vi "Example - Caller is not JKISM++.vi"() -> ()   [LabVIEW 2014]
uses:
  user.lib/_NEVSTOP/JKI State Machine++/AdvanceAPI/CSM - Global Log Event.vi
  user.lib/_NEVSTOP/JKI State Machine++/_Support/JKISMQ/_CSMQFGV.vi
  user.lib/_NEVSTOP/JKI State Machine++/_Support/GlobalEvent/FGV-GlobalEventRef.vi
  user.lib/_NEVSTOP/JKI State Machine++/Communicable State Machine.lvlib
panel:
  in  "Log":bool
  out "Name":string[](array[string])
  in  "DoSth: DoC(error)":bool
  in  "DoSth: DoB":bool
  in  "DoSth: DoA":bool
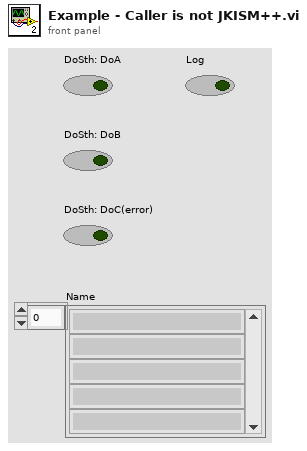
[diagram p1: front panel]
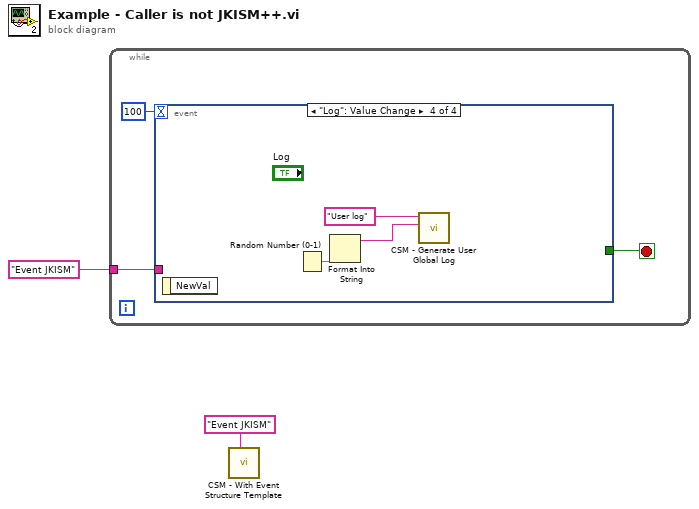
[diagram p0: block diagram]
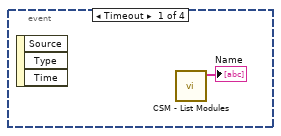
[diagram p2: hidden frame]
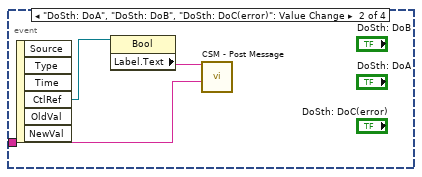
[diagram p3: hidden frame]
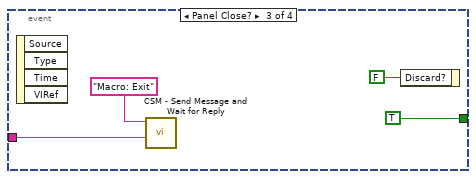
[diagram p4: hidden frame]
diagram:
  n1 = while {
    tunnel: "Event JKISM" ("Name(\"\" to use uuid)") -> [w4]
    stop <- w5 stop-if-true
    n2 = event shown="[3] \"Log\": Value Change" {
      selector: _ -> [_ _ _ _]
      dyn-events: _ -> [_ _ _ _]
      timeout: 100 -> [_ _ _ _]
      tunnel: [_ _ TRUE ("Discard?") _] -> w5
      tunnel: w4 -> [_ w9 w10 _]
      event Timeout {
        n3 = event-data() -> ()  [unwired: 1 in, 3 out]
        n4 = call "CSM - List Modules.vi"() -> ("Module Names"=→"Name":string[])  [unwired: 10 in, 1 out]
      }
      event "DoSth: DoA", "DoSth: DoB", "DoSth: DoC(error)": Value Change {
        n5 = event-data() -> ("CtlRef"=w8:refnum<vi>)  [unwired: 1 in, 5 out]
        n6 = property class="Bool"(reference=w8) -> ("Label.Text"=w7:string)  [unwired: 1 in, 2 out]
        n7 = call "CSM - Post Message.vi"("Target Module"=w9, "State"=w7) -> ()  [unwired: 9 in, 1 out]
      }
      event Panel Close? {
        n8 = event-data() -> ()  [unwired: 1 in, 4 out]
        n9 = call "CSM - Send Message and Wait for Reply.vi"("Target Module"=w10, "State"="Macro: Exit" ("States")) -> ()  [unwired: 8 in, 2 out]
        n10 = event-data("Discard?"=FALSE) -> ()  [unwired: 1 in, 1 out]
      }
      event "Log": Value Change {
        n11 = event-data() -> ()  [unwired: 1 in, 1 out]
        n12 = Random Number (0-1)() -> (number: 0 to 1=w15:dbl)
        n13 = Format Into String(w15) -> (resulting string=w14:string)  [unwired: 3 in, 1 out]
        n14 = call "CSM - Generate User Global Log.vi"("Arguments"=w14, "Log"="User log") -> ()  [unwired: 9 in, 1 out]
      }
    }
  }
  n15 = call "CSM - With Event Structure Template.vi"("Name(\"\" to use uuid)"="Event JKISM" ("Name(\"\" to use uuid)")) -> ()  [unwired: 11 in]
